vi "Analog I_O.vi"() -> ()   [LabVIEW 2025]
panel:
  in  "Pin_AI":u8=32
  out "Valor DAC":u8(knob) scale=0.0..255.0
  in  "Pin_DAC":u8=25 min=25 max=26
  out "Valor DAC":dbl
  in  "stop":bool
  in  "VISA resource name":refnum<visa-resource-name>
  out "error out":errorcluster
  # "Ejemplo: Uso de funciones Analog Read y DAC (Analog Write)\nEste ejemplo muestra cómo utilizar las funciones de adquisición y generación analógica en LV_ESP32.\n\nEntradas requeridas:\nPin_AI: Pin en el que se recibe la señal de voltaje analógico.\nPin_DAC: Pin en el que se generará la señal de salida analógica.\nValor DAC: Valor resultante de la conversión del voltaje de entrada.\n\nSalida generada:\nRepresentación en 8 bits del valor convertido por el DAC."
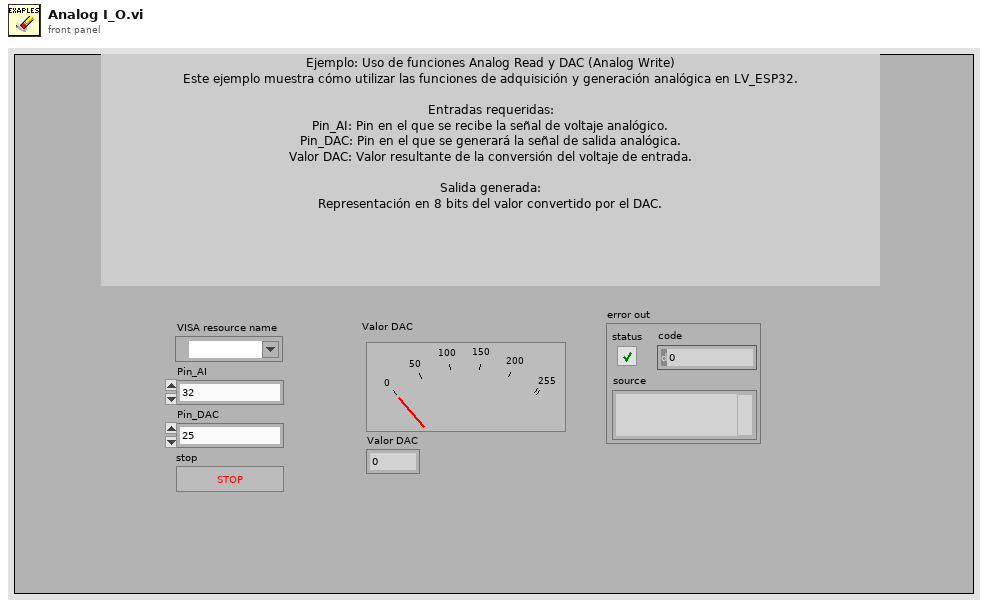
[diagram p1: front panel]
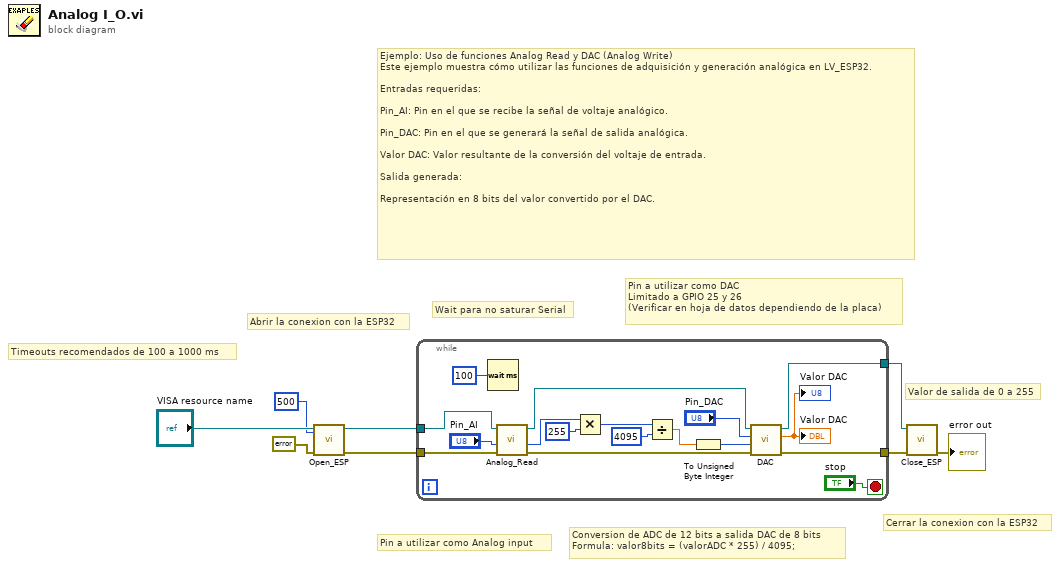
[diagram p0: block diagram]
diagram:
  # "Cerrar la conexion con la ESP32"
  # "Valor de salida de 0 a 255"
  # "Pin a utilizar como DAC\nLimitado a GPIO 25 y 26\n(Verificar en hoja de datos dependiendo de la placa)"
  # "Conversion de ADC de 12 bits a salida DAC de 8 bits\nFormula: valor8bits = (valorADC * 255) / 4095;"
  # "Wait para no saturar Serial"
  # "Pin a utilizar como Analog input"
  # "Timeouts recomendados de 100 a 1000 ms"
  # "Abrir la conexion con la ESP32"
  # "Ejemplo: Uso de funciones Analog Read y DAC (Analog Write)\nEste ejemplo muestra cómo utilizar las funciones de adquisición y generación analógica en LV_ESP32.\n\nEntradas requeridas:\n\nPin_AI: Pin en el que se recibe la señal de voltaje analógico.\n\nPin_DAC: Pin en el que se generará la señal de salida analógica.\n\nValor DAC: Valor resultante de la conversión del voltaje de entrada.\n\nSalida generada:\n\nRepresentación en 8 bits del valor convertido por el DAC."
  n1 = call "Open_ESP.vi"("timeout (10sec)"=u32 500, "error in (no error)"=errorcluster {"status"=FALSE, "code"=0, "source"=""}, "VISA resource name"="VISA resource name") -> ("error out"=w7:errorcluster, "VISA resource name out"=w8:refnum<visa-resource-name>)  [unwired: 7 in]
  n2 = while {
    tunnel: w8 -> [w18]
    tunnel: [w25] -> w6
    tunnel: w7 -> [w19]
    tunnel: [w24] -> w5
    stop <- "stop" stop-if-true
    n3 = Wait (ms)(milliseconds to wait=u32 100) -> ()  [unwired: 1 out]
    n4 = call "Analog_Read.vi"("error in (no error)"=w19, "Pin"="Pin_AI", "VISA resource name"=w18) -> ("error out"=w20:errorcluster, "Analog read"=w16:u16, "VISA resource name out"=w21:refnum<visa-resource-name>)  [unwired: 6 in]
    n5 = Multiply(x=w16, y=255) -> (x*y=w14:i32)
    n6 = Divide(x=w14, y=4095) -> (x/y=w12:dbl)
    n7 = To Unsigned Byte Integer(number=w12) -> (unsigned 8bit integer=w11:u8)
    n8 = call "DAC.vi"("error in (no error)"=w20, "DAC"=w11, "Pin"="Pin_DAC", "VISA resource name"=w21) -> ("error out"=w24:errorcluster, "Voltaje"=→"Valor DAC" →"Valor DAC":dbl, "VISA resource name out"=w25:refnum<visa-resource-name>)  [unwired: 5 in]
  }
  n9 = call "Close_ESP.vi"("error in (no error)"=w5, "VISA resource name"=w6) -> ("error out"=→"error out":errorcluster)  [unwired: 9 in]
